vi "Bus_Monitor_API InitializeSettings.vi"(6 "contextId":T1, 8 "error in":errorcluster, 9 "timeout (ms)":i32=-1, 10 "Request Data":T5, 11 "gRPC ID":T1) -> (0 "error out":errorcluster, 2 "Response Data":T2, 3 "gRPC ID out":T1)   [LabVIEW 2025, in "bus_monitor_client.lvlib"]
uses:
  bus_monitor_client.lvlib
  <vilib>/gRPC/LabVIEW gRPC Library/Shared/grpcId.ctl
  RPC Messages/ni_bus_monitor_api_InitializeSettingsRequest.ctl
  RPC Messages/ni_bus_monitor_api_ConnectSettings.ctl
  RPC Messages/ni_bus_monitor_api_CanMode.ctl
  RPC Messages/ni_bus_monitor_api_Termination.ctl
  RPC Messages/ni_bus_monitor_api_FdIsoMode.ctl
  RPC Messages/ni_bus_monitor_api_InitializeSettingsReply.ctl
  RPC Messages/ni_bus_monitor_api_Session.ctl
  RPC Messages/ni_bus_monitor_api_ErrorInfo.ctl
  RPC Messages/ni_bus_monitor_api_InitializeSettingsReply_Flat.ctl
  RPC Messages/ni_bus_monitor_api_Session_Flat.ctl
  RPC Messages/ni_bus_monitor_api_ErrorInfo_Flat.ctl
  14035477-4c25-4107-8ed5-d0c4ef420ce5.vi
  RPC Messages/RichToFlatni_bus_monitor_api_ConnectSettings.vi
  <vilib>/gRPC/LabVIEW gRPC Library/Shared/TranslateGrpcError.vi
  <vilib>/gRPC/LabVIEW gRPC Library/Shared/Wait On Occurrence.vi
  RPC Messages/FlatToRichni_bus_monitor_api_Session.vi
  RPC Messages/FlatToRichni_bus_monitor_api_ErrorInfo.vi
  <vilib>/gRPC/LabVIEW gRPC Library/Shared/Is Feature Enabled.vi
  <vilib>/gRPC/LabVIEW gRPC Library/Server API/Server/Get Server DLL Path.vi
  <vilib>/Utility/error.llb/Error Cluster From Error Code.vi
  <vilib>/gRPC/LabVIEW gRPC Library/grpc-lvsupport-release.lvlib
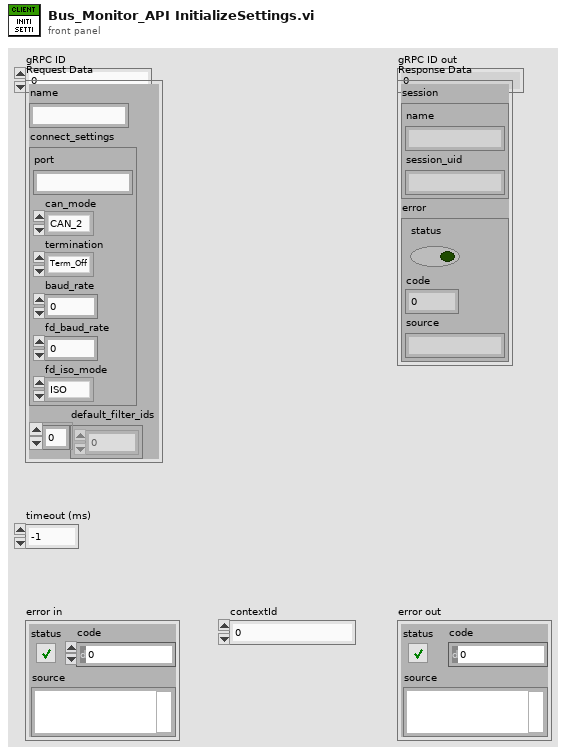
[diagram p1: front panel]
types:
  T1 = typedef "grpc-lvsupport-release.lvlib/grpcId.ctl" = u64
  T2 = typedef "bus_monitor_client.lvlib/ni_bus_monitor_api_InitializeSettingsReply.ctl" = cluster{"session":T3, "error":T4}
  T3 = typedef "bus_monitor_client.lvlib/ni_bus_monitor_api_Session.ctl" = cluster{"name":string, "session_uid":string}
  T4 = typedef "bus_monitor_client.lvlib/ni_bus_monitor_api_ErrorInfo.ctl" = errorcluster
  T5 = typedef "bus_monitor_client.lvlib/ni_bus_monitor_api_InitializeSettingsRequest.ctl" = cluster{"name":string, "connect_settings":T6, "default_filter_ids":u32[]}
  T6 = typedef "bus_monitor_client.lvlib/ni_bus_monitor_api_ConnectSettings.ctl" = cluster{"port":string, "can_mode":T7, "termination":T8, "baud_rate":u64, "fd_baud_rate":u64, "fd_iso_mode":T9}
  T7 = typedef "bus_monitor_client.lvlib/ni_bus_monitor_api_CanMode.ctl" = enum32{"CAN_2", "CAN_FD", "CAN_FD_BRS"}
  T8 = typedef "bus_monitor_client.lvlib/ni_bus_monitor_api_Termination.ctl" = enum32{"Term_Off", "Term_On"}
  T9 = typedef "bus_monitor_client.lvlib/ni_bus_monitor_api_FdIsoMode.ctl" = enum32{"ISO", "Non_ISO", "ISO_Legacy"}
  T10 = typedef "bus_monitor_client.lvlib/ni_bus_monitor_api_InitializeSettingsReply_Flat.ctl" = cluster{"session":T11, "error":T12}
  T11 = typedef "bus_monitor_client.lvlib/ni_bus_monitor_api_Session_Flat.ctl" = cluster{"name":string, "session_uid":string}
  T12 = typedef "bus_monitor_client.lvlib/ni_bus_monitor_api_ErrorInfo_Flat.ctl" = errorcluster
  T13 = typedef "bus_monitor_client.lvlib/ni_bus_monitor_api_InitializeSettingsRequest_Flat.ctl" = cluster{"name":string, "connect_settings":T14, "default_filter_ids":u32[]}
  T14 = typedef "bus_monitor_client.lvlib/ni_bus_monitor_api_ConnectSettings_Flat.ctl" = cluster{"port":string, "can_mode":T7, "termination":T8, "baud_rate":u64, "fd_baud_rate":u64, "fd_iso_mode":T9}
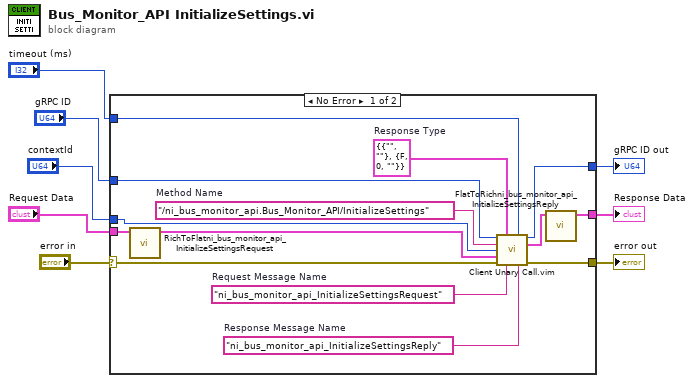
[diagram p0: block diagram]
diagram:
  n1 = case shown="No Error" "error in" {
    selector: "error in" -> [w18 w23]
    tunnel: [w17 w23] -> w7
    tunnel: "gRPC ID" -> [w16 w24]
    tunnel: [w15 w24] -> w5
    tunnel: "Request Data" -> [w12 _]
    tunnel: [w9 _] -> w3
    tunnel: "timeout (ms)" -> [w14 _]
    tunnel: "contextId" -> [w13 _]
    frame No Error {
      w19 = "ni_bus_monitor_api_InitializeSettingsReply"  # Response Message Name
      w20 = "ni_bus_monitor_api_InitializeSettingsRequest"  # Request Message Name
      w21 = T10 {"session"={"name"="", "session_uid"=""}, "error"={"status"=FALSE, "code"=0, "source"=""}}  # Response Type
      w22 = "/ni_bus_monitor_api.Bus_Monitor_API/InitializeSettings"  # Method Name
      n2 = call "RichToFlatni_bus_monitor_api_InitializeSettingsRequest.vi"("InputCluster"=w12) -> ("OutputCluster"=w11:T13)  [unwired: 10 in]
      n3 = call "Client Unary Call.vim"("ClientID in"=w16, "Response Type"=w21, "timeout (ms)"=w14, "Method Name"=w22, "contextId"=w13, "Request Data"=w11, "error in"=w18, "Request Message Name"=w20, "Response Message Name"=w19) -> ("ClientID out"=w15:u64, "Response Data"=w10:T10, "error out"=w17:errorcluster)  [unwired: 4 in]
      n4 = call "FlatToRichni_bus_monitor_api_InitializeSettingsReply.vi"("InputCluster"=w10) -> ("OutputCluster"=w9:T2)  [unwired: 10 in]
    }
    frame Error {
    }
  }
  "error out" <- w7
  "gRPC ID out" <- w5
  "Response Data" <- w3
